vi "220624_TempCalc.vi"(0 "R-Values":dbl[](array[numeric]), 5 "Const. R(0°C)":dbl=100.0, 7 "Const. A":dbl=0.0039, 9 "Const. B":dbl=-5.7e-07) -> (4 "Temp":dbl[](array[numeric]))   [LabVIEW 2021]
uses:
  <vilib>/Utility/error.llb/Error Cluster From Error Code.vi
  <vilib>/ErrorRing/Error Ring.xnode
panel:
  out "error out":errorcluster
  in  "error in (no error)":errorcluster
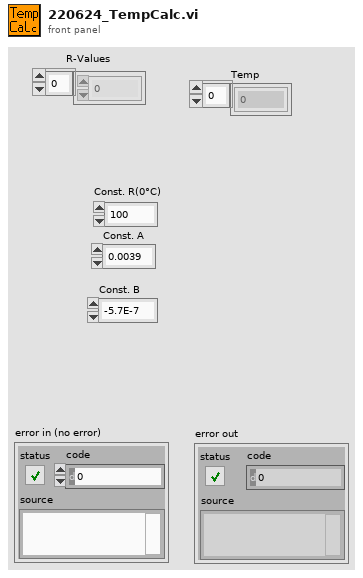
[diagram p1: front panel]
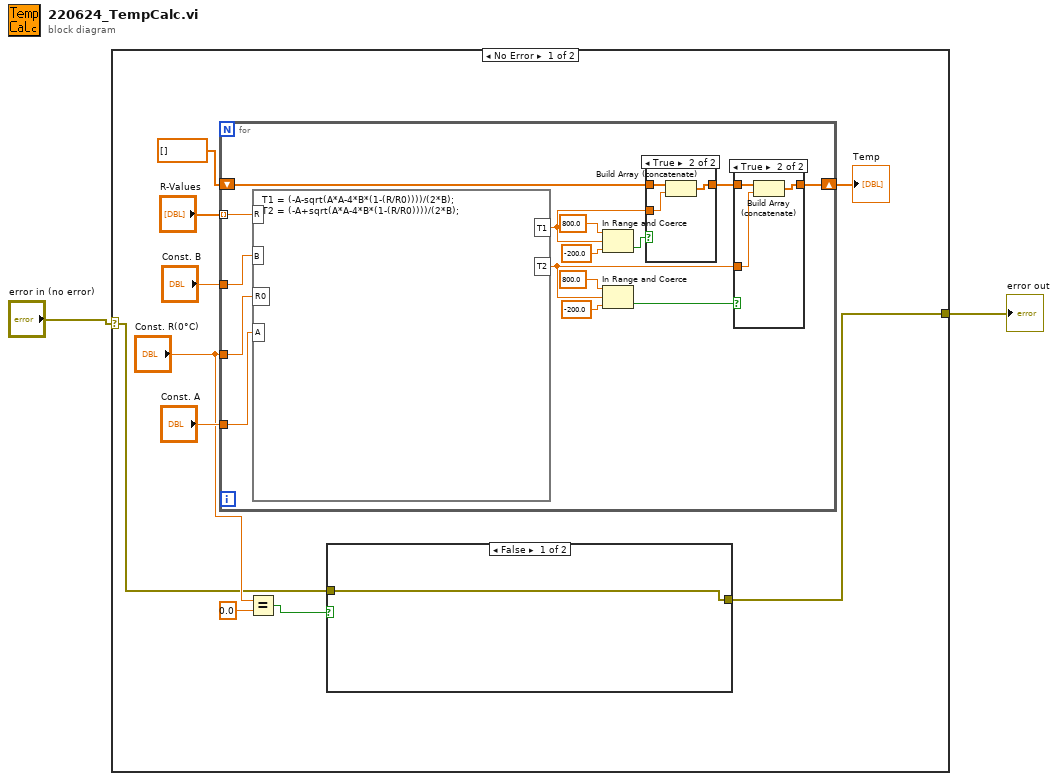
[diagram p0: block diagram]
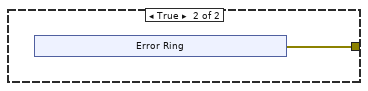
[diagram p2: hidden frame]
diagram:
  n1 = case shown="No Error" "error in (no error)" {
    selector: "error in (no error)" -> [w3 w43]
    tunnel: [w4 w43] -> w1
    frame No Error {
      n2 = for {
        tunnel: "R-Values" -> [w34] mode=indexing
        shift-right: [w25] -> w12
        shift-left: dbl[] [] -> [w24]
        tunnel: "Const. B" -> [w22]
        tunnel: "Const. R(0°C)" -> [w21]
        tunnel: "Const. A" -> [w20]
        n3 = formula code="T1 = (-A-sqrt(A*A-4*B*(1-(R/R0))))/(2*B);\nT2 = (-A+sqrt(A*A-4*B*(1-(R/R0))))/(2*B);"("R"=w34, "B"=w22, "R0"=w21, "A"=w20) -> ("T1"=w28:dbl, "T2"=w26:dbl)
        n4 = In Range and Coerce(upper limit=800.0, x=w28, lower limit=-200.0) -> (In Range?=w29:bool)  [unwired: 1 out]
        n5 = In Range and Coerce(upper limit=800.0, x=w26, lower limit=-200.0) -> (In Range?=w23:bool)  [unwired: 1 out]
        n6 = case shown="True" w29 {
          tunnel: w28 -> [_ w41]
          tunnel: [w39 w42] -> w27
          tunnel: w24 -> [w39 w40]
          frame False {
          }
          frame True {
            n7 = Build Array (concatenate)(w40, w41) -> (w42:dbl[])
          }
        }
        n8 = case shown="True" w23 {
          tunnel: w27 -> [w35 w38]
          tunnel: w26 -> [_ w37]
          tunnel: [w35 w36] -> w25
          frame False {
          }
          frame True {
            n9 = Build Array (concatenate)(w38, w37) -> (w36:dbl[])
          }
        }
      }
      "Temp" <- w12
      n10 = Equal?(x="Const. R(0°C)", y=0.0) -> (x = y?=w5:bool)
      n11 = case shown="False" w5 {
        tunnel: [w13 w14] -> w4
        tunnel: w3 -> [w13 _]
        frame False {
        }
        frame True {
          n12 = xnode "Error Ring"() -> ("error out"=w14:errorcluster)
        }
      }
    }
    frame Error {
    }
  }
  "error out" <- w1
